vi "Run.vi"(8 "error in (no error)":errorcluster, 11 "Project in":refnum<class "Build Job.lvclass">) -> (0 "error out":errorcluster, 2 "Text":string, 3 "Project out":refnum<class "Build Job.lvclass">)   [LabVIEW 2014, in "Build Job.lvclass"]
uses:
  Build Job.lvclass
  Build Job.lvclass/Build Job.ctl
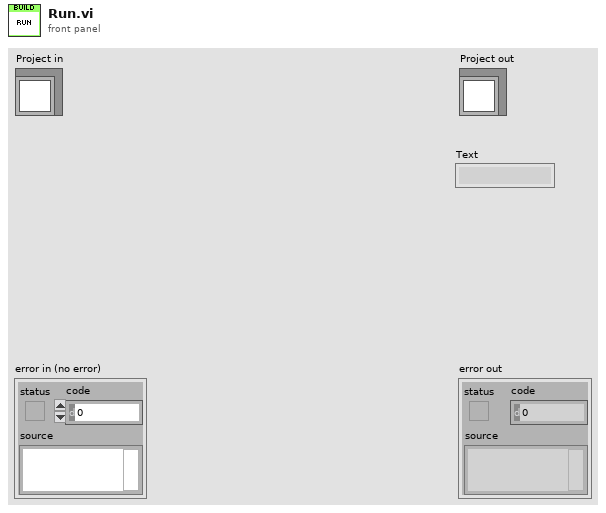
[diagram p1: front panel]
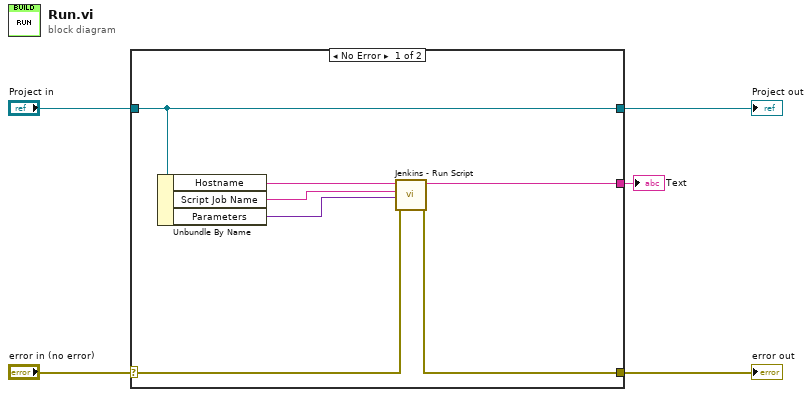
[diagram p0: block diagram]
diagram:
  n1 = case shown="No Error" "error in (no error)" {
    selector: "error in (no error)" -> [w7 w14]
    tunnel: [w6 w14] -> w4
    tunnel: [w12 w13] -> w2
    tunnel: "Project in" -> [w12 w13]
    tunnel: [w8 _] -> w1
    frame No Error {
      n2 = Unbundle By Name(w12) -> ("Hostname"=w11:string, "Script Job Name"=w10:string, "Parameters"=w9:variant)
      n3 = call "Jenkins - Run Script.vi"("error in (no error)"=w7, "Parameters"=w9, "Script Job Name (Within Build Script Folder)"=w10, "IP Address"=w11) -> ("error out"=w6:errorcluster, "Text"=w8:string)  [unwired: 6 in]
    }
    frame Error {
    }
  }
  "error out" <- w4
  "Project out" <- w2
  "Text" <- w1
